vi "Generate Icon Text.vi"(8 "error in (no error)":errorcluster, 11 "Setter Generator In":refnum<class "Setter Generator.lvclass">) -> (0 "error out":errorcluster, 3 "Setter Generator Out":refnum<class "Setter Generator.lvclass">)   [LabVIEW 2020, in "Method Generation.lvlib" / "Setter Generator.lvclass"]
uses:
  Setter Generator.lvclass
  Setter Generator.lvclass/Setter Generator.ctl
  Support/Support.lvlib
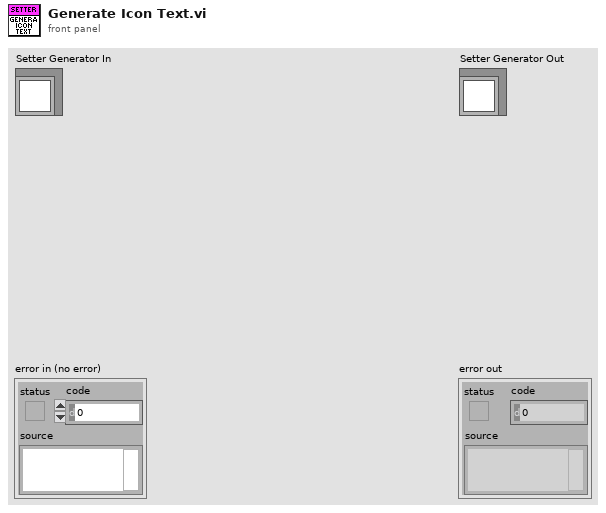
[diagram p1: front panel]
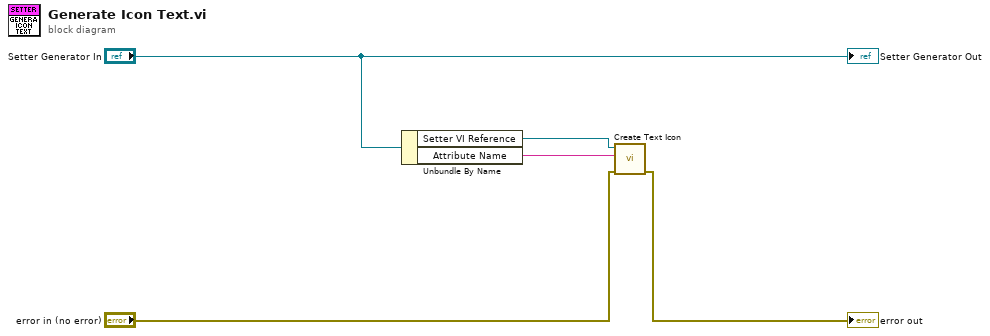
[diagram p0: block diagram]
diagram:
  n1 = Unbundle By Name("Setter Generator In") -> ("Setter VI Reference"=w4:refnum<vi>, "Attribute Name"=w5:string)
  n2 = call "Create Text Icon.vi"("error in (no error)"="error in (no error)", "Icon Text String"=w5, "VI in"=w4) -> ("error out"=→"error out":errorcluster)  [unwired: 7 in, 1 out]
  "Setter Generator Out" <- "Setter Generator In"
